vi "PictureBox.vi"() -> ()   [LabVIEW 2021]
uses:
  System.Windows.Forms
panel:
  out "error out":errorcluster
  in  "Picture Path":path=path "C:/Users/Phalanx/Pictures/Koala.jpg"
  in  "Load":bool
  in  "PictureBox":refnum<k24>(container)
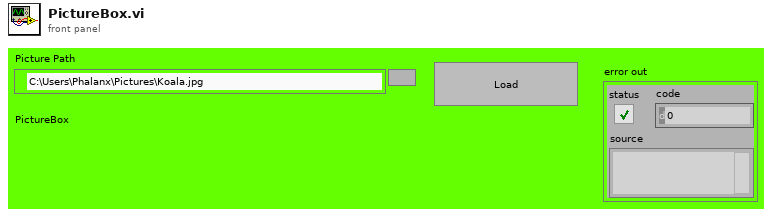
[diagram p1: front panel]
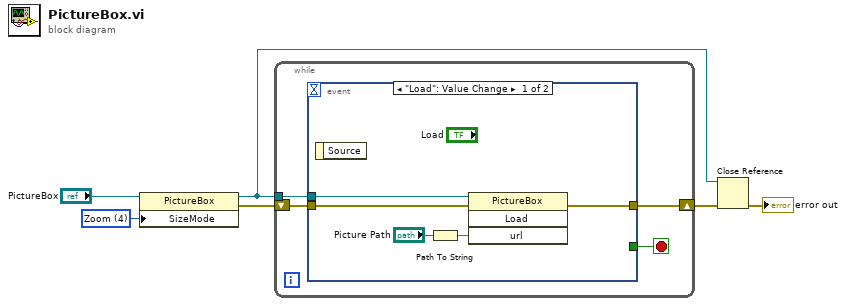
[diagram p0: block diagram]
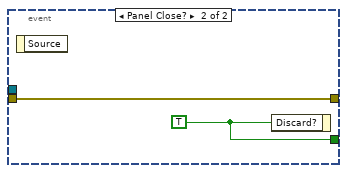
[diagram p2: hidden frame]
diagram:
  w5 = 4 items=["Normal", "StretchImage", "AutoSize", "CenterImage", "Zoom"] ("SizeMode")
  n1 = property class="PictureBox"(reference="PictureBox", "SizeMode"=w5) -> (reference out=w3:refnum<k24>, error out=w4:errorcluster)  [unwired: 1 in]
  n2 = while {
    tunnel: w3 -> [w10]
    shift-right: [w8] -> w2
    shift-left: w4 -> [w7]
    stop <- w9 stop-if-true
    n3 = event shown="[0] \"Load\": Value Change" {
      selector: _ -> [_ _]
      dyn-events: _ -> [_ _]
      timeout: _ -> [_ _]
      tunnel: w10 -> [w15 _]
      tunnel: [_ w17] -> w9
      tunnel: [w12 w16] -> w8
      tunnel: w7 -> [w11 w16]
      event "Load": Value Change {
        n4 = event-data() -> ()  [unwired: 1 in, 1 out]
        n5 = Path To String(path="Picture Path") -> (string=w13:string)
        n6 = invoke class="PictureBox" method="Load"(reference=w15, error in=w11, "url"=w13) -> (error out=w12:errorcluster)  [unwired: 1 in, 3 out]
      }
      event Panel Close? {
        w17 = TRUE
        n7 = event-data() -> ()  [unwired: 1 in, 1 out]
        n8 = event-data("Discard?"=w17) -> ()  [unwired: 1 in, 1 out]
      }
    }
  }
  n9 = Close Reference(reference=w3, error in (no error)=w2) -> (error out=→"error out":errorcluster)
